vi "Untitled 3.vi"(8 "error in (no error)":errorcluster, 11 "GRAFICAR_SEÑAL_ACTUALIZABLE in":refnum<class "GRAFICAR_SEÑAL_ACTUALIZABLE.lvclass">) -> (0 "error out":errorcluster, 3 "GRAFICAR_SEÑAL_ACTUALIZABLE out":refnum<class "GRAFICAR_SEÑAL_ACTUALIZABLE.lvclass">)   [LabVIEW 2019]
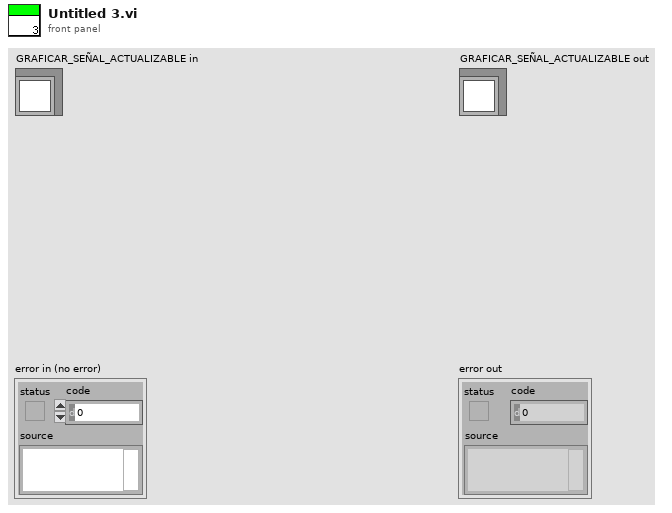
[diagram p1: front panel]
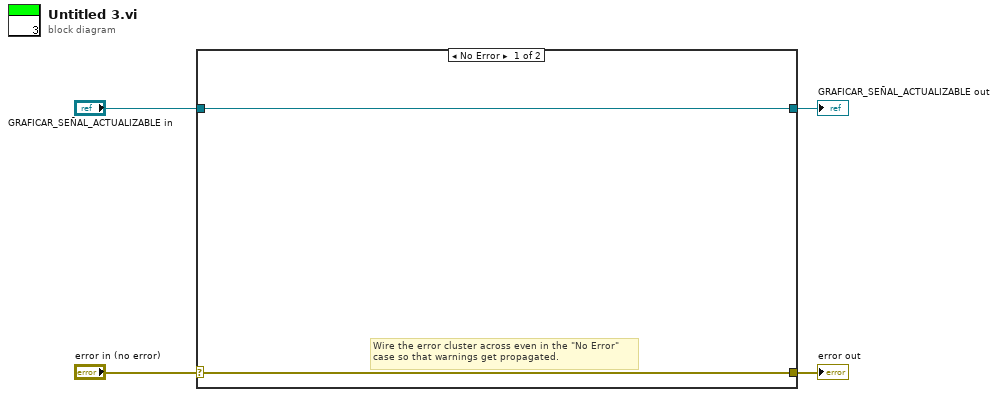
[diagram p0: block diagram]
diagram:
  n1 = case shown="No Error" "error in (no error)" {
    selector: "error in (no error)" -> [w5 w8]
    tunnel: [w5 w8] -> w3
    tunnel: [w6 w7] -> w1
    tunnel: "GRAFICAR_SEÑAL_ACTUALIZABLE in" -> [w6 w7]
    frame No Error {
      # "Wire the error cluster across even in the \"No Error\"\ncase so that warnings get propagated."
    }
    frame Error {
    }
  }
  "error out" <- w3
  "GRAFICAR_SEÑAL_ACTUALIZABLE out" <- w1
